vi "DAQ Clear.vi"(6 "Virtual Dev Error (F)":bool, 8 "error in (no error)":errorcluster, 11 "Refs Data in":T1) -> (0 "error out":errorcluster)   [LabVIEW 2013]
doc: "Usuwa refenencje do sprzêtu pomiarowego"
uses:
  inne pliki/RefData.ctl
  inne pliki/DevSetUp.ctl
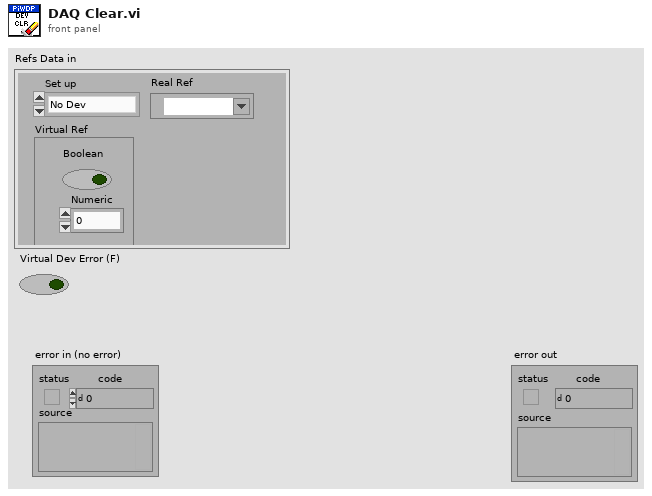
[diagram p1: front panel]
types:
  T1 = typedef "RefData.ctl" = cluster{"Virtual Ref":cluster{"Numeric":dbl, "Boolean":bool}, "Real Ref":refnum<k21>, "Set up":T2}
  T2 = typedef "DevSetUp.ctl" = enum16{"No Dev", "Virtual Dev", "Real Dev"}
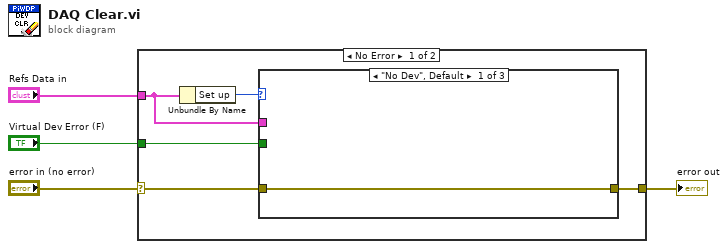
[diagram p0: block diagram]
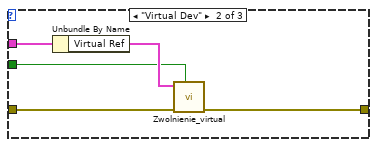
[diagram p2: hidden frame]
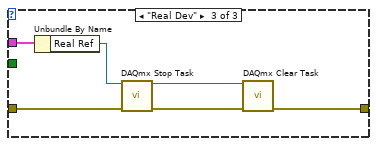
[diagram p3: hidden frame]
diagram:
  n1 = case shown="No Error" "error in (no error)" {
    selector: "error in (no error)" -> [w8 w22]
    tunnel: [w6 w22] -> w3
    tunnel: "Refs Data in" -> [w7 _]
    tunnel: "Virtual Dev Error (F)" -> [w5 _]
    frame No Error {
      n2 = Unbundle By Name(w7) -> ("Set up"=w9:T2)
      n3 = case shown="\"No Dev\", Default" w9 {
        tunnel: w8 -> [w10 w15 w19]
        tunnel: w7 -> [_ w13 w17]
        tunnel: [w10 w12 w18] -> w6
        tunnel: w5 -> [_ w11 _]
        frame "No Dev", Default {
        }
        frame "Virtual Dev" {
          n4 = Unbundle By Name(w13) -> ("Virtual Ref"=w14:cluster{"Numeric":dbl, "Boolean":bool})
          n5 = call "Zwolnienie_virtual.vi"("Error Generate"=w11, "error in (no error)"=w15, "Reference in"=w14) -> ("error out"=w12:errorcluster)  [unwired: 8 in]
        }
        frame "Real Dev" {
          n6 = Unbundle By Name(w17) -> ("Real Ref"=w16:refnum<k21>)
          n7 = call <vilib>:"DAQmx Stop Task.vi"("task/channels in"=w16, "error in"=w19) -> ("task out"=w21:refnum<k21>, "error out"=w20:errorcluster)  [unwired: 12 in]
          n8 = call <vilib>:"DAQmx Clear Task.vi"("task in"=w21, "error in"=w20) -> ("error out"=w18:errorcluster)  [unwired: 13 in]
        }
      }
    }
    frame Error {
    }
  }
  "error out" <- w3
